vi "Get Single Sequence from array.vi"(8 "error in":errorcluster, 10 "TestType":T1, 11 "Sequences":refnum<class "TestSeqClass.lvclass">[](array[class])) -> (0 "error in 2":errorcluster, 2 "Found":bool, 3 "TestSeqClass.lvclass":refnum<class "TestSeqClass.lvclass">)   [LabVIEW 2017]
uses:
  testSeq/TestSeqClass.lvclass
  Typedef/TestTypeSelect.ctl
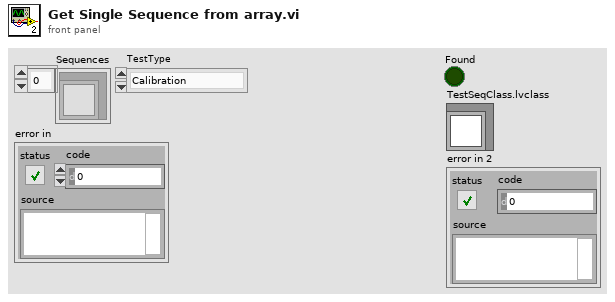
[diagram p1: front panel]
types:
  T1 = typedef "TestTypeSelect.ctl" = enum16{"Calibration", "Testing"}
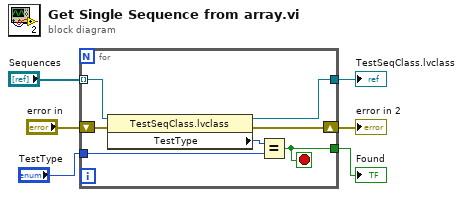
[diagram p0: block diagram]
diagram:
  n1 = for {
    tunnel: "Sequences" -> [w12] mode=indexing
    shift-right: [w10] -> w2
    shift-left: "error in" -> [w11]
    tunnel: [w9] -> w3
    tunnel: [w8] -> w5
    tunnel: "TestType" -> [w7]
    stop <- w8 stop-if-true
    n2 = property class="TestSeqClass.lvclass"(reference=w12, error in=w11) -> (reference out=w9:refnum<class "TestSeqClass.lvclass">, error out=w10:errorcluster, "TestType"=w13:T1)
    n3 = Equal?(x=w13, y=w7) -> (x = y?=w8:bool)
  }
  "Found" <- w5
  "TestSeqClass.lvclass" <- w3
  "error in 2" <- w2
